vi "Sort Combos by Center.vi"() -> ()   [LabVIEW 2023]
panel:
  in  "Circle 2":T1
  in  "Circle 1":T1
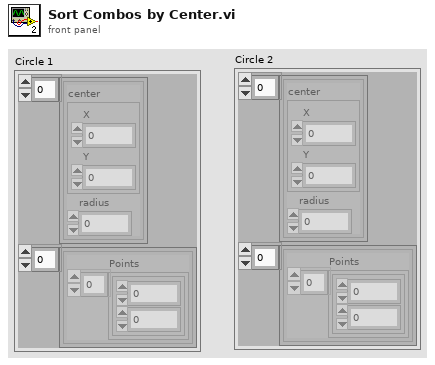
[diagram p1: front panel]
types:
  T1 = cluster{cluster{"center":cluster{"X":sgl, "Y":sgl}, "radius":sgl}[], cluster{"Points":cluster{dbl, dbl}[]}[]}
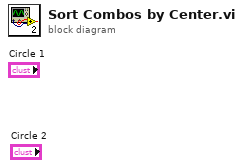
[diagram p0: block diagram]
diagram:
